vi "Grover Search 4.vi"   [LabVIEW 2020]
uses:
  QuSim/Polymorphs/Next_QuVI_Wire.vi
  Gates/Polymorphs/Pauli-X_s.vi
  Gates/Polymorphs/vAControl_e.vi
  Gates/Polymorphs/vAControl_m.vi
  Gates/Polymorphs/vControl_e.vi
  Gates/Polymorphs/vControl_m.vi
  QuSim/Polymorphs/First_QuVI_Wire.vi
  QuSim/QuWire/QuWire.lvclass
panel:
  # "Grover Search Example"
  # "*Open the block diagram for the circuit view (Ctrl+E)"
  # "Performs Grover's Search algorithm to find a marked item in a 4-qubit space (N=16).\n\nThis VI demonstrates amplitude amplification. It uses a 'For Loop' to iterate the Oracle and Diffusion operators approx. 3 times (optimal for N=16). A 'Case Structure' inside allows you to dynamically select which state (e.g., |0101>) is marked by the Oracle. Watch the probability of the target state rise to >96%."
types:
  T1 = enum16{"0000", "0001", "0010", "0011", "0100", "0101", "0110", "0111", "1000", "1001", "1010", "1011", "1100", "1101", "1110", "1111"}
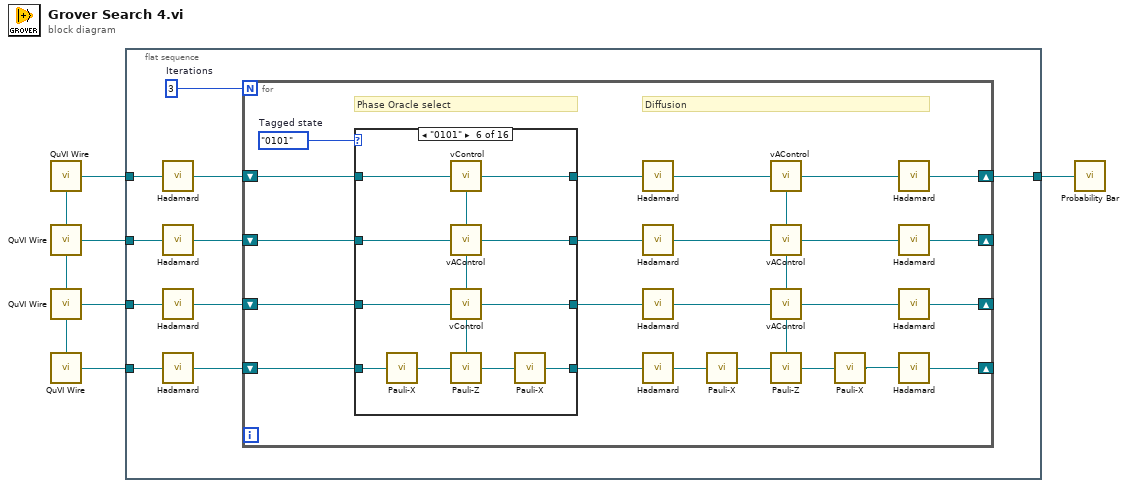
[diagram p0: block diagram]
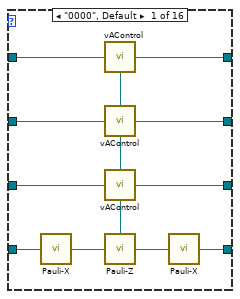
[diagram p2: hidden frame]
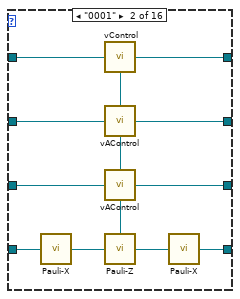
[diagram p3: hidden frame]
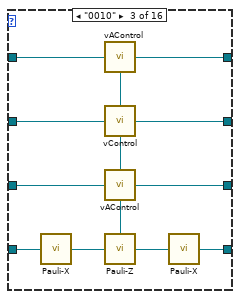
[diagram p4: hidden frame]
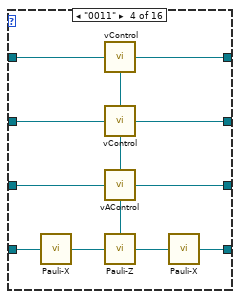
[diagram p5: hidden frame]
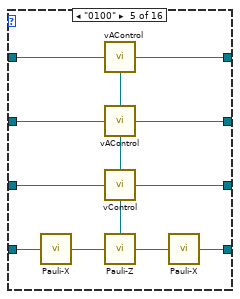
[diagram p6: hidden frame]
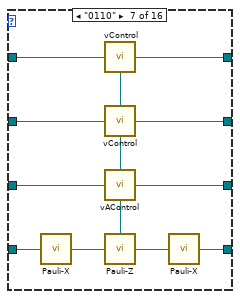
[diagram p7: hidden frame]
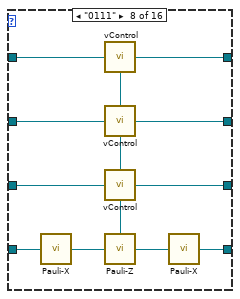
[diagram p8: hidden frame]
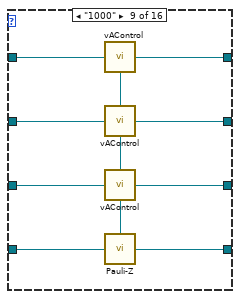
[diagram p9: hidden frame]
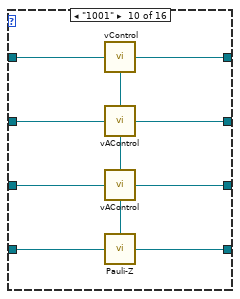
[diagram p10: hidden frame]
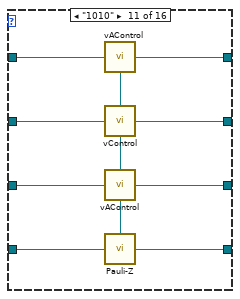
[diagram p11: hidden frame]
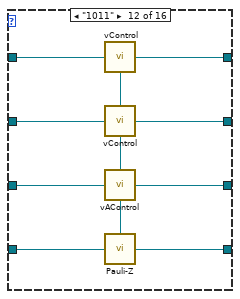
[diagram p12: hidden frame]
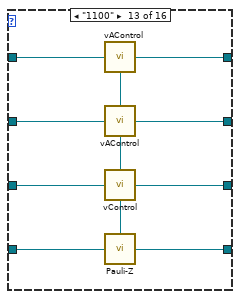
[diagram p13: hidden frame]
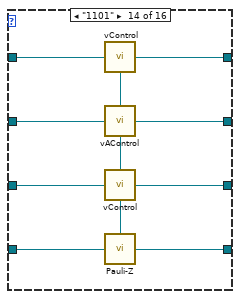
[diagram p14: hidden frame]
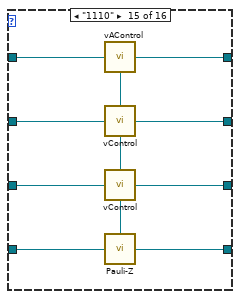
[diagram p15: hidden frame]
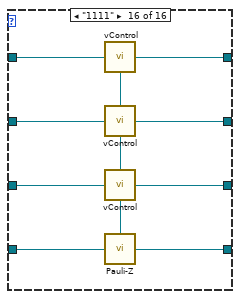
[diagram p16: hidden frame]
diagram:
  n1 = call-poly "QuVI Wire.vi"() -> ("QuVI Wire out"=w6:refnum<class "QuWire.lvclass">, "QuVI out"=w8:refnum<class "QuSim.lvclass">)  [unwired: 14 in]
  n2 = call-poly "QuVI Wire.vi"("QuVI in"=w8) -> ("QuVI Wire out"=w7:refnum<class "QuWire.lvclass">, "QuVI out"=w4:refnum<class "QuSim.lvclass">)  [unwired: 13 in]
  n3 = call-poly "QuVI Wire.vi"("QuVI in"=w4) -> ("QuVI Wire out"=w5:refnum<class "QuWire.lvclass">, "QuVI out"=w2:refnum<class "QuSim.lvclass">)  [unwired: 13 in]
  n4 = call-poly "QuVI Wire.vi"("QuVI in"=w2) -> ("QuVI Wire out"=w3:refnum<class "QuWire.lvclass">)  [unwired: 13 in, 1 out]
  n5 = flat-sequence {
    tunnel: w7 -> [w17]
    tunnel: w6 -> [w18]
    tunnel: w5 -> [w16]
    tunnel: w3 -> [w15]
    tunnel: [w9] -> w1
    frame #0 {
      w14 = 3  # Iterations
      n6 = call "Hadamard.vi"("QuWire in"=w18) -> ("QuWire out"=w11:refnum<class "QuWire.lvclass">)  [unwired: 14 in]
      n7 = call "Hadamard.vi"("QuWire in"=w17) -> ("QuWire out"=w12:refnum<class "QuWire.lvclass">)  [unwired: 14 in]
      n8 = call "Hadamard.vi"("QuWire in"=w16) -> ("QuWire out"=w13:refnum<class "QuWire.lvclass">)  [unwired: 14 in]
      n9 = call "Hadamard.vi"("QuWire in"=w15) -> ("QuWire out"=w10:refnum<class "QuWire.lvclass">)  [unwired: 14 in]
      n10 = for {
        N: w14 -> [_]
        shift-right: [w23] -> w9
        shift-left: w11 -> [w42]
        shift-right: [w20] -> _
        shift-left: w12 -> [w43]
        shift-right: [w22] -> _
        shift-left: w13 -> [w44]
        shift-right: [w19] -> _
        shift-left: w10 -> [w41]
        w21 = T1."0101"  # Tagged state
        # "Phase Oracle select"
        # "Diffusion"
        n11 = case shown="\"0101\"" w21 {
          tunnel: w44 -> [w47 w63 w77 w92 w99 w122 w127 w148 w153 w163 w175 w185 w203 w214 w225 w236]
          tunnel: w43 -> [w57 w70 w72 w86 w109 w121 w124 w138 w159 w170 w176 w186 w202 w213 w220 w228]
          tunnel: w42 -> [w51 w59 w79 w88 w103 w120 w135 w147 w154 w169 w178 w192 w194 w212 w216 w235]
          tunnel: w41 -> [w54 w67 w82 w95 w106 w112 w132 w142 w156 w164 w180 w189 w196 w204 w221 w230]
          tunnel: [w50 w60 w78 w89 w102 w116 w134 w145 w155 w167 w179 w191 w195 w208 w217 w233] -> w40
          tunnel: [w56 w69 w73 w85 w108 w115 w129 w136 w158 w166 w177 w188 w199 w207 w219 w227] -> w39
          tunnel: [w46 w62 w76 w91 w100 w114 w125 w144 w152 w161 w174 w184 w198 w206 w223 w232] -> w38
          tunnel: [w52 w65 w80 w93 w104 w110 w130 w140 w157 w165 w181 w190 w197 w205 w222 w231] -> w37
          frame "0000", Default {
            # "Oracel for 0000 state"
            n12 = call-poly "Pauli-X.vi"("QuWire in"=w54) -> ("QuWire out"=w53:refnum<class "QuWire.lvclass">)  [unwired: 14 in]
            n13 = call-poly "vAControl.vi"("QuWire in"=w51) -> ("QuWire out"=w50:refnum<class "QuWire.lvclass">, "v Ctrl out"=w48:refnum<class "CtrlLine.lvclass">)  [unwired: 13 in]
            n14 = call-poly "vAControl.vi"("v Ctrl in"=w48, "QuWire in"=w57) -> ("QuWire out"=w56:refnum<class "QuWire.lvclass">, "v Ctrl out"=w49:refnum<class "CtrlLine.lvclass">)  [unwired: 12 in]
            n15 = call-poly "vAControl.vi"("v Ctrl in"=w49, "QuWire in"=w47) -> ("QuWire out"=w46:refnum<class "QuWire.lvclass">, "v Ctrl out"=w45:refnum<class "CtrlLine.lvclass">)  [unwired: 12 in]
            n16 = call "Pauli-Z.vi"("v Ctrl in"=w45, "QuWire in"=w53) -> ("QuWire out"=w55:refnum<class "QuWire.lvclass">)  [unwired: 13 in]
            n17 = call-poly "Pauli-X.vi"("QuWire in"=w55) -> ("QuWire out"=w52:refnum<class "QuWire.lvclass">)  [unwired: 14 in]
          }
          frame "0001" {
            # "Oracel for 0001 state"
            n18 = call-poly "Pauli-X.vi"("QuWire in"=w67) -> ("QuWire out"=w66:refnum<class "QuWire.lvclass">)  [unwired: 14 in]
            n19 = call-poly "vControl.vi"("QuWire in"=w59) -> ("QuWire out"=w60:refnum<class "QuWire.lvclass">, "v Ctrl out"=w58:refnum<class "CtrlLine.lvclass">)  [unwired: 13 in]
            n20 = call-poly "vAControl.vi"("v Ctrl in"=w58, "QuWire in"=w70) -> ("QuWire out"=w69:refnum<class "QuWire.lvclass">, "v Ctrl out"=w64:refnum<class "CtrlLine.lvclass">)  [unwired: 12 in]
            n21 = call-poly "vAControl.vi"("v Ctrl in"=w64, "QuWire in"=w63) -> ("QuWire out"=w62:refnum<class "QuWire.lvclass">, "v Ctrl out"=w61:refnum<class "CtrlLine.lvclass">)  [unwired: 12 in]
            n22 = call "Pauli-Z.vi"("v Ctrl in"=w61, "QuWire in"=w66) -> ("QuWire out"=w68:refnum<class "QuWire.lvclass">)  [unwired: 13 in]
            n23 = call-poly "Pauli-X.vi"("QuWire in"=w68) -> ("QuWire out"=w65:refnum<class "QuWire.lvclass">)  [unwired: 14 in]
          }
          frame "0010" {
            # "Oracel for 0010 state"
            n24 = call-poly "Pauli-X.vi"("QuWire in"=w82) -> ("QuWire out"=w81:refnum<class "QuWire.lvclass">)  [unwired: 14 in]
            n25 = call-poly "vAControl.vi"("QuWire in"=w79) -> ("QuWire out"=w78:refnum<class "QuWire.lvclass">, "v Ctrl out"=w74:refnum<class "CtrlLine.lvclass">)  [unwired: 13 in]
            n26 = call-poly "vControl.vi"("v Ctrl in"=w74, "QuWire in"=w72) -> ("QuWire out"=w73:refnum<class "QuWire.lvclass">, "v Ctrl out"=w71:refnum<class "CtrlLine.lvclass">)  [unwired: 12 in]
            n27 = call-poly "vAControl.vi"("v Ctrl in"=w71, "QuWire in"=w77) -> ("QuWire out"=w76:refnum<class "QuWire.lvclass">, "v Ctrl out"=w75:refnum<class "CtrlLine.lvclass">)  [unwired: 12 in]
            n28 = call "Pauli-Z.vi"("v Ctrl in"=w75, "QuWire in"=w81) -> ("QuWire out"=w83:refnum<class "QuWire.lvclass">)  [unwired: 13 in]
            n29 = call-poly "Pauli-X.vi"("QuWire in"=w83) -> ("QuWire out"=w80:refnum<class "QuWire.lvclass">)  [unwired: 14 in]
          }
          frame "0011" {
            # "Oracel for 0011 state"
            n30 = call-poly "Pauli-X.vi"("QuWire in"=w95) -> ("QuWire out"=w94:refnum<class "QuWire.lvclass">)  [unwired: 14 in]
            n31 = call-poly "vControl.vi"("QuWire in"=w88) -> ("QuWire out"=w89:refnum<class "QuWire.lvclass">, "v Ctrl out"=w87:refnum<class "CtrlLine.lvclass">)  [unwired: 13 in]
            n32 = call-poly "vControl.vi"("v Ctrl in"=w87, "QuWire in"=w86) -> ("QuWire out"=w85:refnum<class "QuWire.lvclass">, "v Ctrl out"=w84:refnum<class "CtrlLine.lvclass">)  [unwired: 12 in]
            n33 = call-poly "vAControl.vi"("v Ctrl in"=w84, "QuWire in"=w92) -> ("QuWire out"=w91:refnum<class "QuWire.lvclass">, "v Ctrl out"=w90:refnum<class "CtrlLine.lvclass">)  [unwired: 12 in]
            n34 = call "Pauli-Z.vi"("v Ctrl in"=w90, "QuWire in"=w94) -> ("QuWire out"=w96:refnum<class "QuWire.lvclass">)  [unwired: 13 in]
            n35 = call-poly "Pauli-X.vi"("QuWire in"=w96) -> ("QuWire out"=w93:refnum<class "QuWire.lvclass">)  [unwired: 14 in]
          }
          frame "0100" {
            # "Oracel for 0100 state"
            n36 = call-poly "Pauli-X.vi"("QuWire in"=w106) -> ("QuWire out"=w105:refnum<class "QuWire.lvclass">)  [unwired: 14 in]
            n37 = call-poly "vAControl.vi"("QuWire in"=w103) -> ("QuWire out"=w102:refnum<class "QuWire.lvclass">, "v Ctrl out"=w101:refnum<class "CtrlLine.lvclass">)  [unwired: 13 in]
            n38 = call-poly "vAControl.vi"("v Ctrl in"=w101, "QuWire in"=w109) -> ("QuWire out"=w108:refnum<class "QuWire.lvclass">, "v Ctrl out"=w97:refnum<class "CtrlLine.lvclass">)  [unwired: 12 in]
            n39 = call-poly "vControl.vi"("v Ctrl in"=w97, "QuWire in"=w99) -> ("QuWire out"=w100:refnum<class "QuWire.lvclass">, "v Ctrl out"=w98:refnum<class "CtrlLine.lvclass">)  [unwired: 12 in]
            n40 = call "Pauli-Z.vi"("v Ctrl in"=w98, "QuWire in"=w105) -> ("QuWire out"=w107:refnum<class "QuWire.lvclass">)  [unwired: 13 in]
            n41 = call-poly "Pauli-X.vi"("QuWire in"=w107) -> ("QuWire out"=w104:refnum<class "QuWire.lvclass">)  [unwired: 14 in]
          }
          frame "0101" {
            # "Oracel for 0101 state"
            n42 = call-poly "Pauli-X.vi"("QuWire in"=w112) -> ("QuWire out"=w111:refnum<class "QuWire.lvclass">)  [unwired: 14 in]
            n43 = call-poly "vControl.vi"("QuWire in"=w120) -> ("QuWire out"=w116:refnum<class "QuWire.lvclass">, "v Ctrl out"=w119:refnum<class "CtrlLine.lvclass">)  [unwired: 13 in]
            n44 = call-poly "vAControl.vi"("v Ctrl in"=w119, "QuWire in"=w121) -> ("QuWire out"=w115:refnum<class "QuWire.lvclass">, "v Ctrl out"=w118:refnum<class "CtrlLine.lvclass">)  [unwired: 12 in]
            n45 = call-poly "vControl.vi"("v Ctrl in"=w118, "QuWire in"=w122) -> ("QuWire out"=w114:refnum<class "QuWire.lvclass">, "v Ctrl out"=w117:refnum<class "CtrlLine.lvclass">)  [unwired: 12 in]
            n46 = call "Pauli-Z.vi"("v Ctrl in"=w117, "QuWire in"=w111) -> ("QuWire out"=w113:refnum<class "QuWire.lvclass">)  [unwired: 13 in]
            n47 = call-poly "Pauli-X.vi"("QuWire in"=w113) -> ("QuWire out"=w110:refnum<class "QuWire.lvclass">)  [unwired: 14 in]
          }
          frame "0110" {
            # "Oracel for 0110 state"
            n48 = call-poly "Pauli-X.vi"("QuWire in"=w132) -> ("QuWire out"=w131:refnum<class "QuWire.lvclass">)  [unwired: 14 in]
            n49 = call-poly "vControl.vi"("QuWire in"=w135) -> ("QuWire out"=w134:refnum<class "QuWire.lvclass">, "v Ctrl out"=w128:refnum<class "CtrlLine.lvclass">)  [unwired: 13 in]
            n50 = call-poly "vControl.vi"("v Ctrl in"=w128, "QuWire in"=w124) -> ("QuWire out"=w129:refnum<class "QuWire.lvclass">, "v Ctrl out"=w123:refnum<class "CtrlLine.lvclass">)  [unwired: 12 in]
            n51 = call-poly "vAControl.vi"("v Ctrl in"=w123, "QuWire in"=w127) -> ("QuWire out"=w125:refnum<class "QuWire.lvclass">, "v Ctrl out"=w126:refnum<class "CtrlLine.lvclass">)  [unwired: 12 in]
            n52 = call "Pauli-Z.vi"("v Ctrl in"=w126, "QuWire in"=w131) -> ("QuWire out"=w133:refnum<class "QuWire.lvclass">)  [unwired: 13 in]
            n53 = call-poly "Pauli-X.vi"("QuWire in"=w133) -> ("QuWire out"=w130:refnum<class "QuWire.lvclass">)  [unwired: 14 in]
          }
          frame "0111" {
            # "Oracel for 0111 state"
            n54 = call-poly "Pauli-X.vi"("QuWire in"=w142) -> ("QuWire out"=w141:refnum<class "QuWire.lvclass">)  [unwired: 14 in]
            n55 = call-poly "vControl.vi"("QuWire in"=w147) -> ("QuWire out"=w145:refnum<class "QuWire.lvclass">, "v Ctrl out"=w139:refnum<class "CtrlLine.lvclass">)  [unwired: 13 in]
            n56 = call-poly "vControl.vi"("v Ctrl in"=w139, "QuWire in"=w138) -> ("QuWire out"=w136:refnum<class "QuWire.lvclass">, "v Ctrl out"=w137:refnum<class "CtrlLine.lvclass">)  [unwired: 12 in]
            n57 = call-poly "vControl.vi"("v Ctrl in"=w137, "QuWire in"=w148) -> ("QuWire out"=w144:refnum<class "QuWire.lvclass">, "v Ctrl out"=w146:refnum<class "CtrlLine.lvclass">)  [unwired: 12 in]
            n58 = call "Pauli-Z.vi"("v Ctrl in"=w146, "QuWire in"=w141) -> ("QuWire out"=w143:refnum<class "QuWire.lvclass">)  [unwired: 13 in]
            n59 = call-poly "Pauli-X.vi"("QuWire in"=w143) -> ("QuWire out"=w140:refnum<class "QuWire.lvclass">)  [unwired: 14 in]
          }
          frame "1000" {
            # "Oracel for 1 state"
            n60 = call-poly "vAControl.vi"("QuWire in"=w154) -> ("QuWire out"=w155:refnum<class "QuWire.lvclass">, "v Ctrl out"=w149:refnum<class "CtrlLine.lvclass">)  [unwired: 13 in]
            n61 = call-poly "vAControl.vi"("v Ctrl in"=w149, "QuWire in"=w159) -> ("QuWire out"=w158:refnum<class "QuWire.lvclass">, "v Ctrl out"=w150:refnum<class "CtrlLine.lvclass">)  [unwired: 12 in]
            n62 = call-poly "vAControl.vi"("v Ctrl in"=w150, "QuWire in"=w153) -> ("QuWire out"=w152:refnum<class "QuWire.lvclass">, "v Ctrl out"=w151:refnum<class "CtrlLine.lvclass">)  [unwired: 12 in]
            n63 = call "Pauli-Z.vi"("v Ctrl in"=w151, "QuWire in"=w156) -> ("QuWire out"=w157:refnum<class "QuWire.lvclass">)  [unwired: 13 in]
          }
          frame "1001" {
            # "Oracel for 0101 state"
            n64 = call-poly "vControl.vi"("QuWire in"=w169) -> ("QuWire out"=w167:refnum<class "QuWire.lvclass">, "v Ctrl out"=w168:refnum<class "CtrlLine.lvclass">)  [unwired: 13 in]
            n65 = call-poly "vAControl.vi"("v Ctrl in"=w168, "QuWire in"=w170) -> ("QuWire out"=w166:refnum<class "QuWire.lvclass">, "v Ctrl out"=w162:refnum<class "CtrlLine.lvclass">)  [unwired: 12 in]
            n66 = call-poly "vAControl.vi"("v Ctrl in"=w162, "QuWire in"=w163) -> ("QuWire out"=w161:refnum<class "QuWire.lvclass">, "v Ctrl out"=w160:refnum<class "CtrlLine.lvclass">)  [unwired: 12 in]
            n67 = call "Pauli-Z.vi"("v Ctrl in"=w160, "QuWire in"=w164) -> ("QuWire out"=w165:refnum<class "QuWire.lvclass">)  [unwired: 13 in]
          }
          frame "1010" {
            # "Oracel for 0101 state"
            n68 = call-poly "vAControl.vi"("QuWire in"=w178) -> ("QuWire out"=w179:refnum<class "QuWire.lvclass">, "v Ctrl out"=w171:refnum<class "CtrlLine.lvclass">)  [unwired: 13 in]
            n69 = call-poly "vControl.vi"("v Ctrl in"=w171, "QuWire in"=w176) -> ("QuWire out"=w177:refnum<class "QuWire.lvclass">, "v Ctrl out"=w172:refnum<class "CtrlLine.lvclass">)  [unwired: 12 in]
            n70 = call-poly "vAControl.vi"("v Ctrl in"=w172, "QuWire in"=w175) -> ("QuWire out"=w174:refnum<class "QuWire.lvclass">, "v Ctrl out"=w173:refnum<class "CtrlLine.lvclass">)  [unwired: 12 in]
            n71 = call "Pauli-Z.vi"("v Ctrl in"=w173, "QuWire in"=w180) -> ("QuWire out"=w181:refnum<class "QuWire.lvclass">)  [unwired: 13 in]
          }
          frame "1011" {
            # "Oracel for 0101 state"
            n72 = call-poly "vControl.vi"("QuWire in"=w192) -> ("QuWire out"=w191:refnum<class "QuWire.lvclass">, "v Ctrl out"=w187:refnum<class "CtrlLine.lvclass">)  [unwired: 13 in]
            n73 = call-poly "vControl.vi"("v Ctrl in"=w187, "QuWire in"=w186) -> ("QuWire out"=w188:refnum<class "QuWire.lvclass">, "v Ctrl out"=w182:refnum<class "CtrlLine.lvclass">)  [unwired: 12 in]
            n74 = call-poly "vAControl.vi"("v Ctrl in"=w182, "QuWire in"=w185) -> ("QuWire out"=w184:refnum<class "QuWire.lvclass">, "v Ctrl out"=w183:refnum<class "CtrlLine.lvclass">)  [unwired: 12 in]
            n75 = call "Pauli-Z.vi"("v Ctrl in"=w183, "QuWire in"=w189) -> ("QuWire out"=w190:refnum<class "QuWire.lvclass">)  [unwired: 13 in]
          }
          frame "1100" {
            # "Oracel for 0101 state"
            n76 = call-poly "vAControl.vi"("QuWire in"=w194) -> ("QuWire out"=w195:refnum<class "QuWire.lvclass">, "v Ctrl out"=w193:refnum<class "CtrlLine.lvclass">)  [unwired: 13 in]
            n77 = call-poly "vAControl.vi"("v Ctrl in"=w193, "QuWire in"=w202) -> ("QuWire out"=w199:refnum<class "QuWire.lvclass">, "v Ctrl out"=w201:refnum<class "CtrlLine.lvclass">)  [unwired: 12 in]
            n78 = call-poly "vControl.vi"("v Ctrl in"=w201, "QuWire in"=w203) -> ("QuWire out"=w198:refnum<class "QuWire.lvclass">, "v Ctrl out"=w200:refnum<class "CtrlLine.lvclass">)  [unwired: 12 in]
            n79 = call "Pauli-Z.vi"("v Ctrl in"=w200, "QuWire in"=w196) -> ("QuWire out"=w197:refnum<class "QuWire.lvclass">)  [unwired: 13 in]
          }
          frame "1101" {
            # "Oracel for 0101 state"
            n80 = call-poly "vControl.vi"("QuWire in"=w212) -> ("QuWire out"=w208:refnum<class "QuWire.lvclass">, "v Ctrl out"=w211:refnum<class "CtrlLine.lvclass">)  [unwired: 13 in]
            n81 = call-poly "vAControl.vi"("v Ctrl in"=w211, "QuWire in"=w213) -> ("QuWire out"=w207:refnum<class "QuWire.lvclass">, "v Ctrl out"=w210:refnum<class "CtrlLine.lvclass">)  [unwired: 12 in]
            n82 = call-poly "vControl.vi"("v Ctrl in"=w210, "QuWire in"=w214) -> ("QuWire out"=w206:refnum<class "QuWire.lvclass">, "v Ctrl out"=w209:refnum<class "CtrlLine.lvclass">)  [unwired: 12 in]
            n83 = call "Pauli-Z.vi"("v Ctrl in"=w209, "QuWire in"=w204) -> ("QuWire out"=w205:refnum<class "QuWire.lvclass">)  [unwired: 13 in]
          }
          frame "1110" {
            # "Oracel for 0101 state"
            n84 = call-poly "vAControl.vi"("QuWire in"=w216) -> ("QuWire out"=w217:refnum<class "QuWire.lvclass">, "v Ctrl out"=w218:refnum<class "CtrlLine.lvclass">)  [unwired: 13 in]
            n85 = call-poly "vControl.vi"("v Ctrl in"=w218, "QuWire in"=w220) -> ("QuWire out"=w219:refnum<class "QuWire.lvclass">, "v Ctrl out"=w215:refnum<class "CtrlLine.lvclass">)  [unwired: 12 in]
            n86 = call-poly "vControl.vi"("v Ctrl in"=w215, "QuWire in"=w225) -> ("QuWire out"=w223:refnum<class "QuWire.lvclass">, "v Ctrl out"=w224:refnum<class "CtrlLine.lvclass">)  [unwired: 12 in]
            n87 = call "Pauli-Z.vi"("v Ctrl in"=w224, "QuWire in"=w221) -> ("QuWire out"=w222:refnum<class "QuWire.lvclass">)  [unwired: 13 in]
          }
          frame "1111" {
            # "Oracel for 0101 state"
            n88 = call-poly "vControl.vi"("QuWire in"=w235) -> ("QuWire out"=w233:refnum<class "QuWire.lvclass">, "v Ctrl out"=w229:refnum<class "CtrlLine.lvclass">)  [unwired: 13 in]
            n89 = call-poly "vControl.vi"("v Ctrl in"=w229, "QuWire in"=w228) -> ("QuWire out"=w227:refnum<class "QuWire.lvclass">, "v Ctrl out"=w226:refnum<class "CtrlLine.lvclass">)  [unwired: 12 in]
            n90 = call-poly "vControl.vi"("v Ctrl in"=w226, "QuWire in"=w236) -> ("QuWire out"=w232:refnum<class "QuWire.lvclass">, "v Ctrl out"=w234:refnum<class "CtrlLine.lvclass">)  [unwired: 12 in]
            n91 = call "Pauli-Z.vi"("v Ctrl in"=w234, "QuWire in"=w230) -> ("QuWire out"=w231:refnum<class "QuWire.lvclass">)  [unwired: 13 in]
          }
        }
        n92 = call "Hadamard.vi"("QuWire in"=w40) -> ("QuWire out"=w36:refnum<class "QuWire.lvclass">)  [unwired: 14 in]
        n93 = call "Hadamard.vi"("QuWire in"=w39) -> ("QuWire out"=w34:refnum<class "QuWire.lvclass">)  [unwired: 14 in]
        n94 = call "Hadamard.vi"("QuWire in"=w38) -> ("QuWire out"=w35:refnum<class "QuWire.lvclass">)  [unwired: 14 in]
        n95 = call "Hadamard.vi"("QuWire in"=w37) -> ("QuWire out"=w28:refnum<class "QuWire.lvclass">)  [unwired: 14 in]
        n96 = call-poly "Pauli-X.vi"("QuWire in"=w28) -> ("QuWire out"=w27:refnum<class "QuWire.lvclass">)  [unwired: 14 in]
        n97 = call-poly "vAControl.vi"("QuWire in"=w36) -> ("QuWire out"=w33:refnum<class "QuWire.lvclass">, "v Ctrl out"=w30:refnum<class "CtrlLine.lvclass">)  [unwired: 13 in]
        n98 = call-poly "vAControl.vi"("v Ctrl in"=w30, "QuWire in"=w34) -> ("QuWire out"=w32:refnum<class "QuWire.lvclass">, "v Ctrl out"=w31:refnum<class "CtrlLine.lvclass">)  [unwired: 12 in]
        n99 = call-poly "vAControl.vi"("v Ctrl in"=w31, "QuWire in"=w35) -> ("QuWire out"=w29:refnum<class "QuWire.lvclass">, "v Ctrl out"=w24:refnum<class "CtrlLine.lvclass">)  [unwired: 12 in]
        n100 = call "Pauli-Z.vi"("v Ctrl in"=w24, "QuWire in"=w27) -> ("QuWire out"=w26:refnum<class "QuWire.lvclass">)  [unwired: 13 in]
        n101 = call-poly "Pauli-X.vi"("QuWire in"=w26) -> ("QuWire out"=w25:refnum<class "QuWire.lvclass">)  [unwired: 14 in]
        n102 = call "Hadamard.vi"("QuWire in"=w33) -> ("QuWire out"=w23:refnum<class "QuWire.lvclass">)  [unwired: 14 in]
        n103 = call "Hadamard.vi"("QuWire in"=w32) -> ("QuWire out"=w20:refnum<class "QuWire.lvclass">)  [unwired: 14 in]
        n104 = call "Hadamard.vi"("QuWire in"=w29) -> ("QuWire out"=w22:refnum<class "QuWire.lvclass">)  [unwired: 14 in]
        n105 = call "Hadamard.vi"("QuWire in"=w25) -> ("QuWire out"=w19:refnum<class "QuWire.lvclass">)  [unwired: 14 in]
      }
    }
  }
  n106 = call "Probability Bar.vi"("QuWire in"=w1) -> ()  [unwired: 13 in, 2 out]
